vi "SerialCharWRtermchar.vi"(0 "VISA resource name":refnum<visa-resource-name>="COM8", 1 "baud rate":u32=115200, 2 "data bits":u16=8 min=5 max=8 step=1, 3 "parity":u16(ring) items=["None", "Odd", "Even", "Mark", "Space"], 4 "stop bits":u16(ring)=10 items=["1.0"=10, "1.5"=15, "2.0"=20], 7 "flow control":u16(ring) items=["None"=0, "XON/XOFF"=1, "RTS/CTS"=2, "DTR/DSR"=4], 10 "write buffer":string) -> (5 "#bytes read":u32, 6 "error?":bool, 9 "read buffer":string)   [LabVIEW 2012]
doc: "The Basic Serial Read and Write example performs a Serial Port Read, a Serial Port Write, or a combination of these actions. The user selects the actions (read or write) on the front panel. If both are selected, the VI will write the data first, read data, and then close the VISA session that is opened to the port. This VI will wait until the specified number of bytes is received at the port. Only the number of bytes specified will be read.\n\nINSTRUCTIONS:\n1) Select the serial resource and configuration parameters (baud rate, data bits, parity, stop bits, flow control).\n2) Select the operations to be performed. \n3) Connect the serial port to your device. If no device is available, perform a loopback test by doing one of the following. Short pins 2 and 3 on a RS-232 cable or short pin 4 to pin 8 and pin 5 to pin 9 on a RS-485/422 cable. \n4) Run the VI to see the data read. (The \"read string\" will match the \"string to write\" if a loopback test was performed.)\n\nNote: The parameters set for the serial port must match the parameters of the connected instrument or device. In this example, the bytes to read parameter specifies the number of bytes that the serial port reads. If there were more bytes at the port than the number specified in bytes to read, those bytes would not be read. Also, if you specify to read more bytes than the number of bytes actually read, you might receive a timeout error message.\n\nOn the block diagram, the Configure Serial Port VI sets the configuration parameters. The front panel displays the controls used to configure the basic parameters, such as baud rate, data bits, and parity. Constants configure the other parameters the user probably does not need set. After the VISA Configure Serial Port VI opens the VISA session and configures the port, the VI passes the VISA resource name to other VIs that perform operations on that VISA resource. The VISA Write function sends a command to the serial device and the VISA Read function returns data based on the command. The VISA Close function then closes the reference to the serial device. It is important to close the reference; otherwise communication through with that port through protocols other than VISA might not be possible."
uses:
  <vilib>/Utility/error.llb/DialogType.ctl
  <vilib>/Instr/_visa.llb/VISA Configure Serial Port (Instr).vi
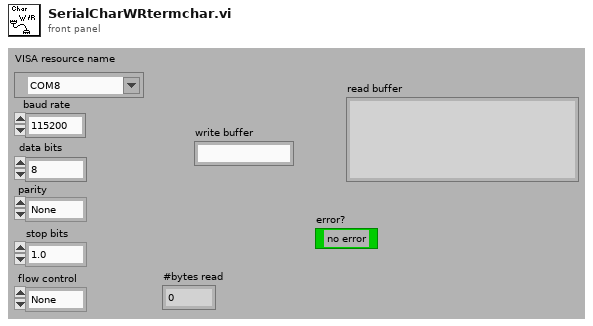
[diagram p1: front panel]
types:
  T1 = typedef "DialogType.ctl" = u16
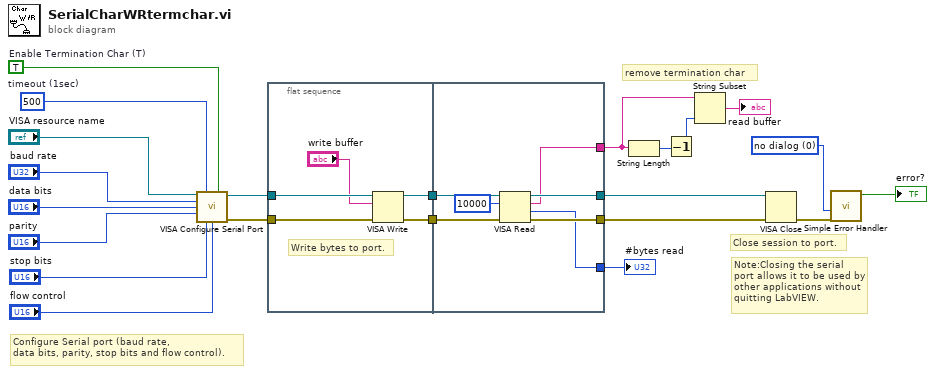
[diagram p0: block diagram]
diagram:
  w9 = T1 0 items=["no dialog", "OK message", "continue or stop message", "OK message + warnings", "continue/stop + warnings"] ("type of dialog (OK msg:1)")
  w15 = TRUE  # Enable Termination Char (T)
  w16 = u32 500  # timeout (1sec)
  # "remove termination char"
  # "Note:Closing the serial port allows it to be used by other applications without\nquitting LabVIEW."
  # "Configure Serial port (baud rate,\ndata bits, parity, stop bits and flow control)."
  # "Close session to port."
  n1 = call-poly "VISA Configure Serial Port"("VISA resource name"="VISA resource name", "timeout (10sec)"=w16, "Enable Termination\nChar (T)"=w15, "baud rate (9600)"="baud rate", "data bits (8)"="data bits", "parity (0:none)"="parity", "stop bits (10: 1 bit)"="stop bits", "flow control (0:none)"="flow control") -> ("VISA resource name out"=w19:refnum<visa-resource-name>, "error out"=w20:errorcluster)  [unwired: 1 in, 5 out]
  n2 = flat-sequence {
    tunnel: w20 -> [w27]
    tunnel: w19 -> [w26]
    tunnel: [w24] -> w6
    tunnel: [w23] -> w5
    tunnel: [w34] -> w11
    tunnel: [w33] -> w10
    tunnel: [w32] -> w7
    tunnel: w6 -> [w31]
    tunnel: w5 -> [w30]
    tunnel: [w28] -> w4
    frame #0 {
      # "Write bytes to port."
      n3 = VISA Write(VISA resource name=w26, write buffer="write buffer", error in (no error)=w27) -> (VISA resource name out=w24:refnum<visa-resource-name>, error out=w23:errorcluster)  [unwired: 1 out]
    }
    frame #1 {
      n4 = VISA Read(VISA resource name=w31, byte count=u32 10000, error in (no error)=w30) -> (VISA resource name out=w33:refnum<visa-resource-name>, read buffer=w28:string, return count=w32:u32, error out=w34:errorcluster)
    }
  }
  n5 = String Length(string=w4) -> (length=w2:i32)
  n6 = Decrement(x=w2) -> (x-1=w1:i32)
  n7 = String Subset(string=w4, length (rest)=w1) -> (substring=→"read buffer":string)  [unwired: 1 in]
  n8 = VISA Close(VISA resource name=w10, error in (no error)=w11) -> (error out=w18:errorcluster)
  n9 = call <vilib>:"Simple Error Handler.vi"("type of dialog (OK msg:1)"=w9, "error in (no error)"=w18) -> ("error?"=→"error?":bool)  [unwired: 7 out]
  "#bytes read" <- w7
